vi "Update_Events.vi"(8 "Status/Errors in":refnum<vi>, 9 "Events for screen":refnum<queue>, 10 "Control Parameters [] in":T15[](array[typedef]) {"Aux Byte Value" format="%02x"; "Max Real Value" format="%#_6e"; "Min Real Value" format="%#_6e"; "dReal/dByte" format="%#_6e"; "Byte Value" format="%02x"; "Identifier" format="%02x"}, 11 "Main parameters in":T1={"Mode"={"Mode"=enum."Dialog", "Expert?"=FALSE, "Dialog?"=FALSE}, "Stop loop"={"Settings changed?"=FALSE, "Stop?"=refnum}, "Send message"={"Send mode"=enum."Get parameters", "Set parameter list"=0, "Get parameter list"=0, "Reset device"=0, "Length set settings message"=0, "Reset buttons?"=FALSE, "Reset Master?"=enum."General"}, "Write settings"={"Options"=enum."File 1"}, "Settings state"={"MAS locked?"=refnum, "SLV locked?"=refnum}, "Button refs"={"Stop program"=refnum, "Save settings"=refnum, "DAQ mode"=refnum, "Reset settings"=refnum, "Apply settings"=refnum, "Reset MAS"=refnum, "Reset SLV"=refnum, "Local DBase?"=refnum, "Last value DBase"=FALSE, "Database"=refnum, "Calibration"=refnum, "Save settings 2"=refnum}, "Update screen"={"Detector number"=0, "Hardware"=enum."None"}, "Files"={"Path config file"=path "", "Path def. ini file"=path "", "Path ini file 1"=path "", "Path ini file 2"=path "", "Path RBF file"=path ""}, "DB connection"={"connection reference"=refnum, "Connected?"=refnum, "ODBC Name"=""}, "Status_id"=refnum, "Time difference"=refnum, "Satellites"=refnum, "Alignment parameters"=refnum, "Page Statistics 2"=refnum, "Database"=refnum, "Page Statistics"=refnum} {"Update screen"."Detector number" format="%#.0f"; "Send message"."Reset device" format="%x"; "Send message"."Get parameter list" format="%x"; "Send message"."Set parameter list" format="%x"}) -> (0 "Status/Errors out":refnum<vi>, 2 "Control Parameters [] out":T15[](array[typedef]) {"Aux Byte Value" format="%02x"; "Max Real Value" format="%#_6e"; "Min Real Value" format="%#_6e"; "dReal/dByte" format="%#_6e"; "Byte Value" format="%02x"; "Identifier" format="%02x"}, 3 "Main parameters out":T1={"Mode"={"Mode"=enum."Dialog", "Expert?"=FALSE, "Dialog?"=FALSE}, "Stop loop"={"Settings changed?"=FALSE, "Stop?"=refnum}, "Send message"={"Send mode"=enum."Get parameters", "Set parameter list"=0, "Get parameter list"=0, "Reset device"=0, "Length set settings message"=0, "Reset buttons?"=FALSE, "Reset Master?"=enum."General"}, "Write settings"={"Options"=enum."File 1"}, "Settings state"={"MAS locked?"=refnum, "SLV locked?"=refnum}, "Button refs"={"Stop program"=refnum, "Save settings"=refnum, "DAQ mode"=refnum, "Reset settings"=refnum, "Apply settings"=refnum, "Reset MAS"=refnum, "Reset SLV"=refnum, "Local DBase?"=refnum, "Last value DBase"=FALSE, "Database"=refnum, "Calibration"=refnum, "Save settings 2"=refnum}, "Update screen"={"Detector number"=0, "Hardware"=enum."None"}, "Files"={"Path config file"=path "", "Path def. ini file"=path "", "Path ini file 1"=path "", "Path ini file 2"=path "", "Path RBF file"=path ""}, "DB connection"={"connection reference"=refnum, "Connected?"=refnum, "ODBC Name"=""}, "Status_id"=refnum, "Time difference"=refnum, "Satellites"=refnum, "Alignment parameters"=refnum, "Page Statistics 2"=refnum, "Database"=refnum, "Page Statistics"=refnum} {"Update screen"."Detector number" format="%#.0f"; "Send message"."Reset device" format="%x"; "Send message"."Get parameter list" format="%x"; "Send message"."Set parameter list" format="%x"}, 4 "Updated?":bool)   [LabVIEW 2013]
uses:
  Controls/Control_Parameters.ctl
  Controls/Master.ctl
  Controls/Main_Parameters.ctl
  Controls/Mode.ctl
  Controls/Stop_Loop.ctl
  Controls/Send_Message.ctl
  Controls/Send_Message_Mode.ctl
  Controls/Write_Settings.ctl
  Controls/Write_Settings_Options.ctl
  Controls/Settings_State.ctl
  Controls/Button_Refs.ctl
  Controls/Update_Screen.ctl
  Controls/Files.ctl
  Controls/DB_Connection.ctl
  database/Connection.llb/Conn ObjectReference.ctl
  Controls/Status_Errors_Elements.ctl
  Controls/Get_Set_Statistics_Options2.ctl
  Controls/TabPage_Events.ctl
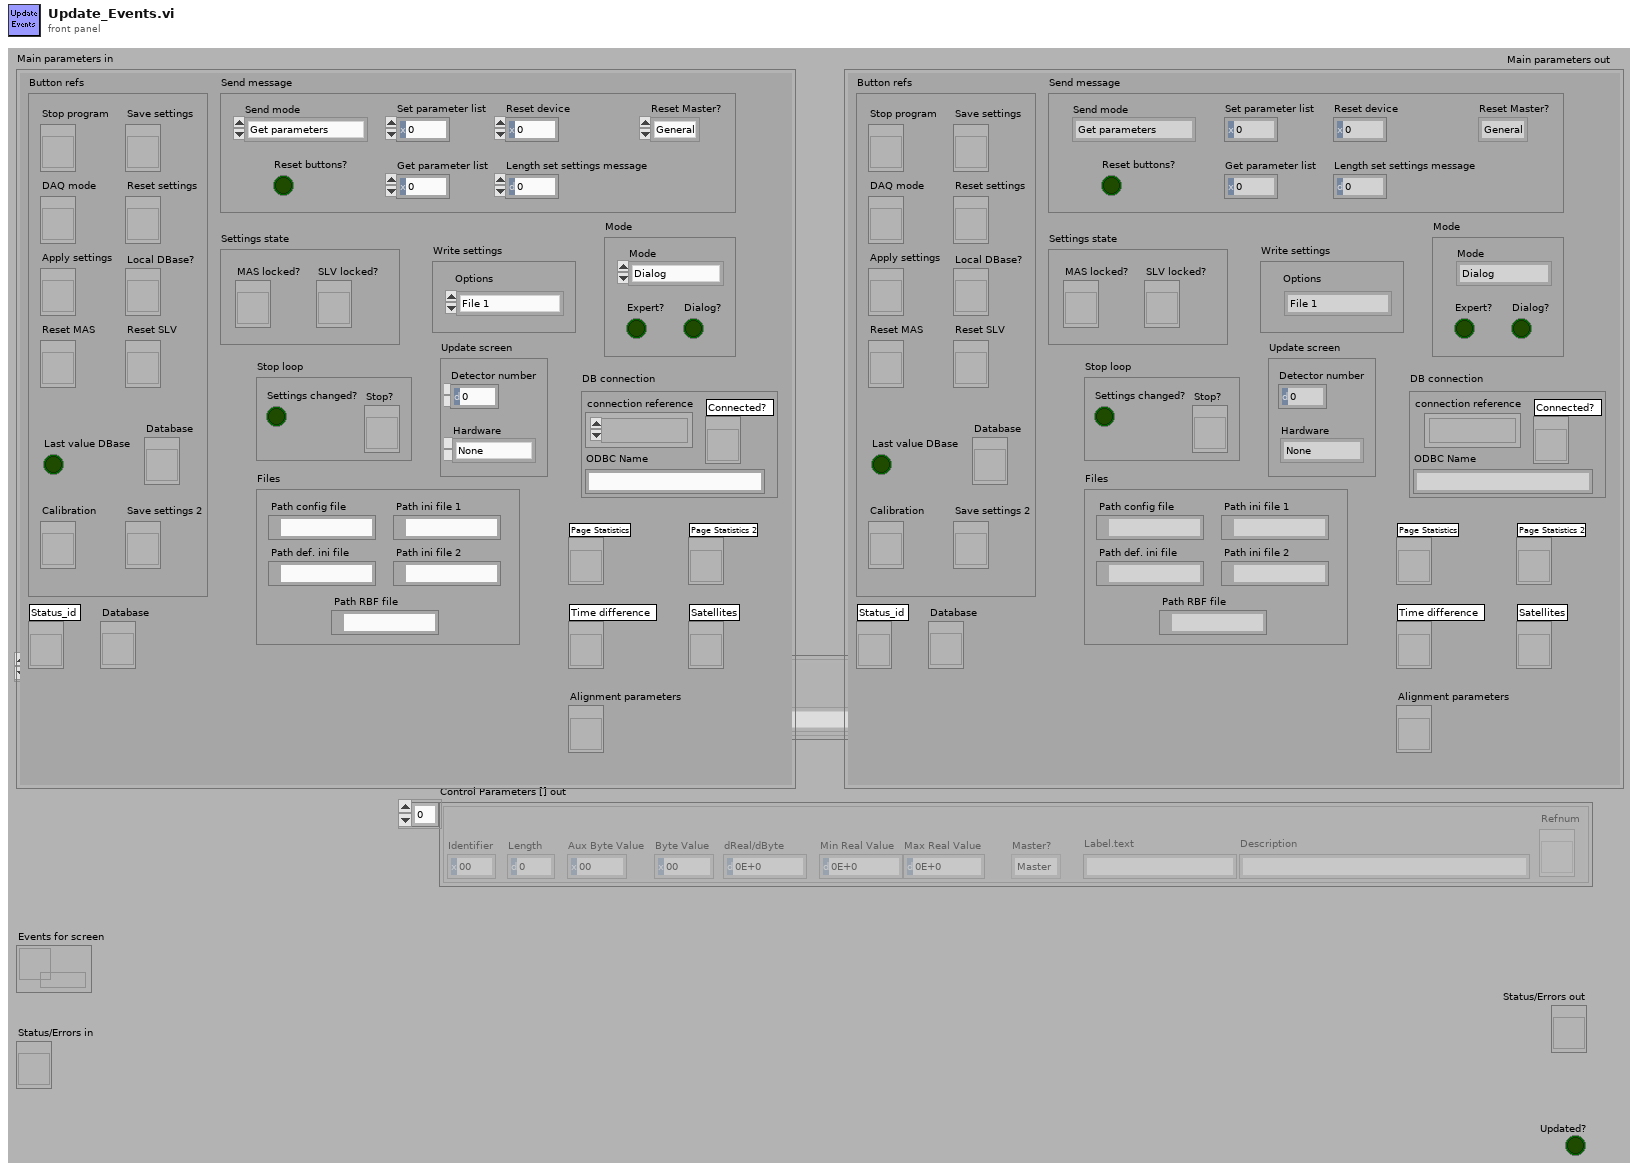
[diagram p1: front panel]
types:
  T1 = typedef "Main_Parameters.ctl" = cluster{"Mode":T2, "Stop loop":T3, "Send message":T4, "Write settings":T7, "Settings state":T9, "Button refs":T10, "Update screen":T11, "Files":T12, "DB connection":T13, "Status_id":refnum<vi>, "Time difference":refnum<vi>, "Satellites":refnum<vi>, "Alignment parameters":refnum<vi>, "Page Statistics 2":refnum<vi>, "Database":refnum<vi>, "Page Statistics":refnum<vi>}
  T2 = typedef "Mode.ctl" = cluster{"Mode":enum8{"Stop", "Dialog", "Hisparc II", "Hisparc II DAQ", "Alignment"}, "Expert?":bool, "Dialog?":bool}
  T3 = typedef "Stop_Loop.ctl" = cluster{"Settings changed?":bool, "Stop?":refnum<vi>}
  T4 = typedef "Send_Message.ctl" = cluster{"Send mode":T5, "Set parameter list":u8, "Get parameter list":u8, "Reset device":u8, "Length set settings message":i32, "Reset buttons?":bool, "Reset Master?":T6}
  T5 = typedef "Send_Message_Mode.ctl" = enum16{"Get parameters", "Set parameters", "From front panel", "From parameters", "Reset device", "Alignment"}
  T6 = typedef "Master.ctl" = enum16{"Master", "Slave", "General"}
  T7 = typedef "Write_Settings.ctl" = cluster{"Options":T8}
  T8 = typedef "Write_Settings_Options.ctl" = enum16{"File 1", "File 2", "Alignment", "Reset"}
  T9 = typedef "Settings_State.ctl" = cluster{"MAS locked?":refnum<vi>, "SLV locked?":refnum<vi>}
  T10 = typedef "Button_Refs.ctl" = cluster{"Stop program":refnum<vi>, "Save settings":refnum<vi>, "DAQ mode":refnum<vi>, "Reset settings":refnum<vi>, "Apply settings":refnum<vi>, "Reset MAS":refnum<vi>, "Reset SLV":refnum<vi>, "Local DBase?":refnum<vi>, "Last value DBase":bool, "Database":refnum<vi>, "Calibration":refnum<vi>, "Save settings 2":refnum<vi>}
  T11 = typedef "Update_Screen.ctl" = cluster{"Detector number":u16, "Hardware":enum8{"None", "HiSPARC I", "HiSPARC II", "HiSPARC III", "Unknown"}}
  T12 = typedef "Files.ctl" = cluster{"Path config file":path, "Path def. ini file":path, "Path ini file 1":path, "Path ini file 2":path, "Path RBF file":path}
  T13 = typedef "DB_Connection.ctl" = cluster{"connection reference":T14, "Connected?":refnum<vi>, "ODBC Name":string}
  T14 = typedef "Conn ObjectReference.ctl" = refnum<k1>
  T15 = typedef "Control_Parameters.ctl" = cluster{"Identifier":u8, "Length":u16, "Byte Value":u32, "dReal/dByte":dbl, "Min Real Value":dbl, "Max Real Value":dbl, "Master?":T6, "Label.text":string, "Description":string, "Refnum":refnum<vi>, "Aux Byte Value":u32}
  T16 = typedef "TabPage_Events.ctl" = cluster{"Det_Numb":u16, "GPS_Timestamp":string, "Trigger_Pattern":cluster{"Master ch. 1 lower threshold":bool, "Master ch. 1 higher threshold":bool, "Master ch. 2 lower threshold":bool, "Master ch. 2 higher threshold":bool, "Slave ch. 1 lower threshold":bool, "Slave ch. 1 higher threshold":bool, "Slave ch. 2 lower threshold":bool, "Slave ch. 2 higher threshold":bool, "External trigger":bool, "Slave present?":bool, "Ch. 1 low comparator master":bool, "Ch. 1 high comparator master":bool, "Ch. 2 low comparator master":bool, "Ch. 2 high comparator master":bool, "Ch. 1 low comparator slave":bool, "Ch. 1 high comparator slave":bool, "Ch. 2 low comparator slave":bool, "Ch. 2 high comparator slave":bool}, "Traces":dbl[][], "MAS_Status_Events":bool, "MAS_Vers_Numb":string, "SLV_Status_Events":bool, "SLV_Vers_Numb":string, "DBase_connected?":bool, "MAS_GPS_Long":dbl, "MAS_GPS_Lat":dbl, "MAS_GPS_Alt":dbl, "Hardware":enum8{"None", "HiSPARC I", "HiSPARC II", "HiSPARC III", "Unknown"}}
  T17 = typedef "Get_Set_Statistics_Options2.ctl" = enum16{"Get", "Set"}
  T18 = typedef "Status_Errors_Elements.ctl" = enum16{"Default", "Errors", "Master status", "Slave status", "Master connected?", "Slave connected?", "Master GPS on board?", "Slave GPS on board?", "Master: slave detected?", "Slave: slave detected?", "Last message from master", "Last message from slave", "Master temperature", "GPS settings correct?"}
  T19 = typedef "Event_Statistics.ctl" = cluster{"Baseline 1":i16, "Baseline 2":i16, "Number of peaks 1":i16, "Number of peaks 2":i16, "Pulse height 1":i16, "Pulse height 2":i16, "Integral 1":i32, "Integral 2":i32, "Standard deviation 1":i16, "Standard deviation 2":i16, "Length":i32, "Time difference":u32}
  T20 = cluster{"Master ch. 1 lower threshold":bool, "Master ch. 1 higher threshold":bool, "Master ch. 2 lower threshold":bool, "Master ch. 2 higher threshold":bool, "Slave ch. 1 lower threshold":bool, "Slave ch. 1 higher threshold":bool, "Slave ch. 2 lower threshold":bool, "Slave ch. 2 higher threshold":bool, "External trigger":bool, "Slave present?":bool, "Ch. 1 low comparator master":bool, "Ch. 1 high comparator master":bool, "Ch. 2 low comparator master":bool, "Ch. 2 high comparator master":bool, "Ch. 1 low comparator slave":bool, "Ch. 1 high comparator slave":bool, "Ch. 2 low comparator slave":bool, "Ch. 2 high comparator slave":bool}
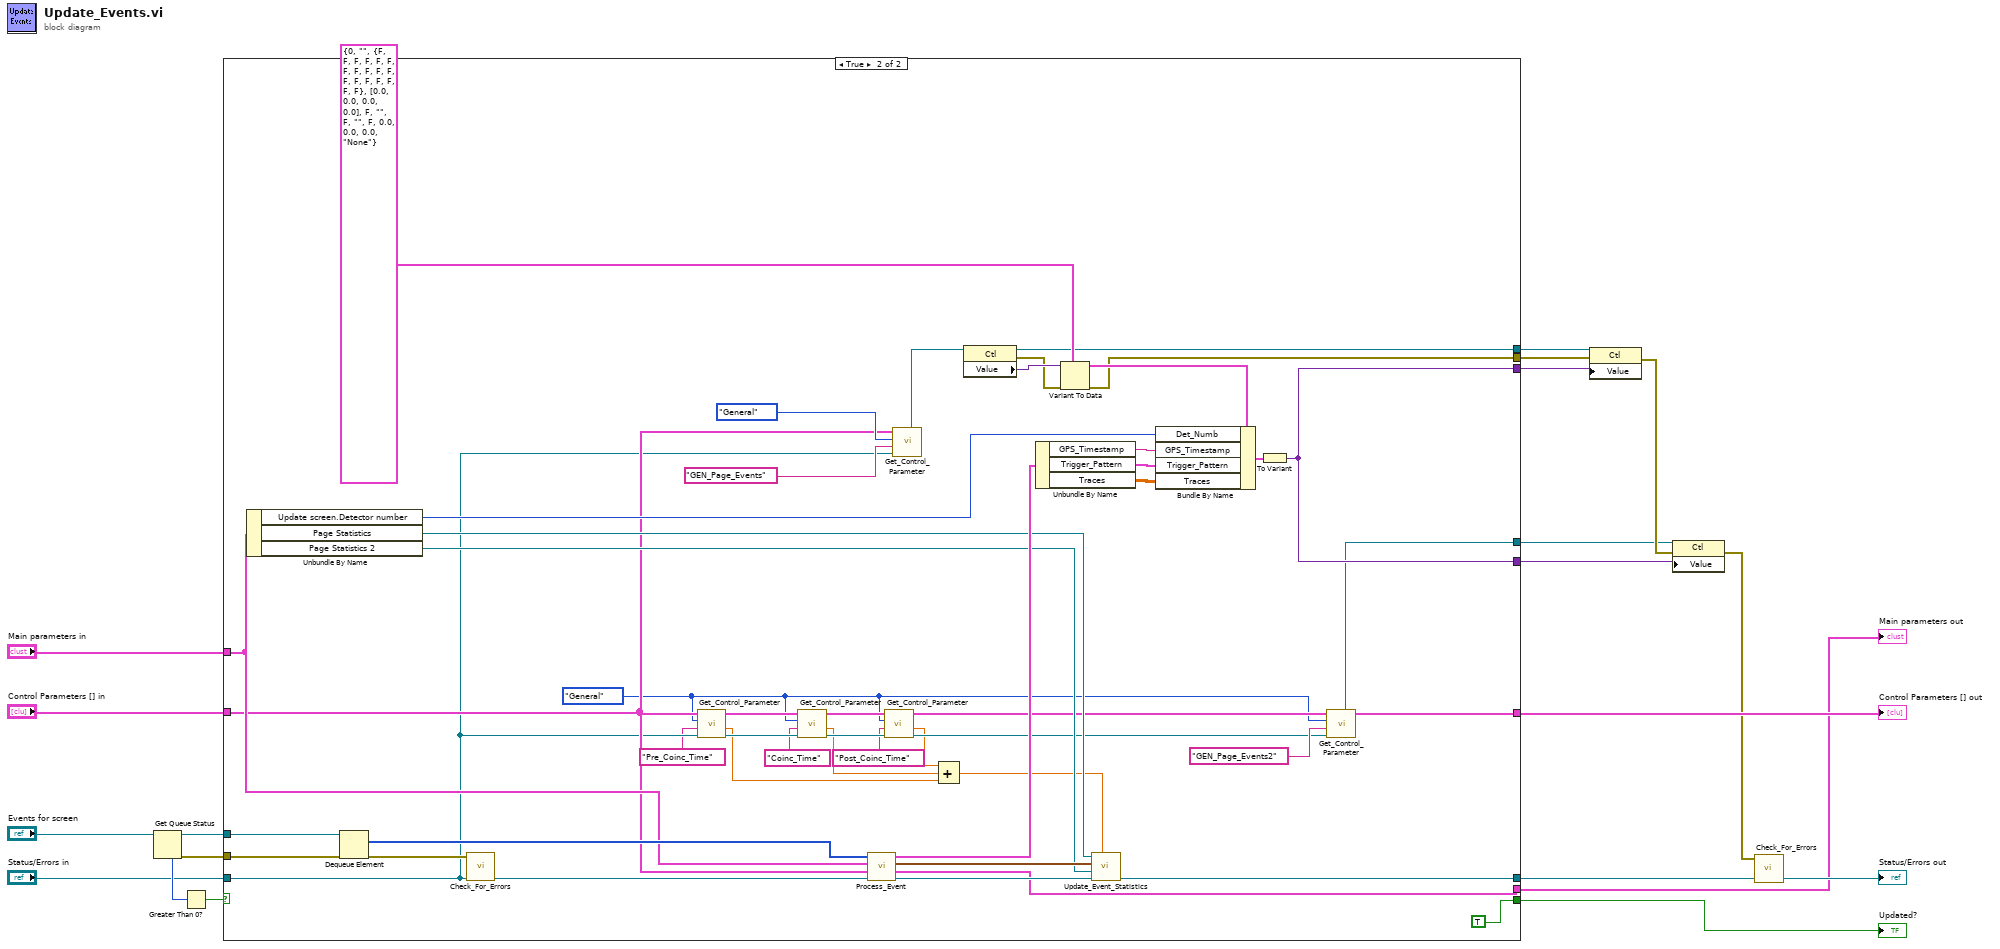
[diagram p0: block diagram]
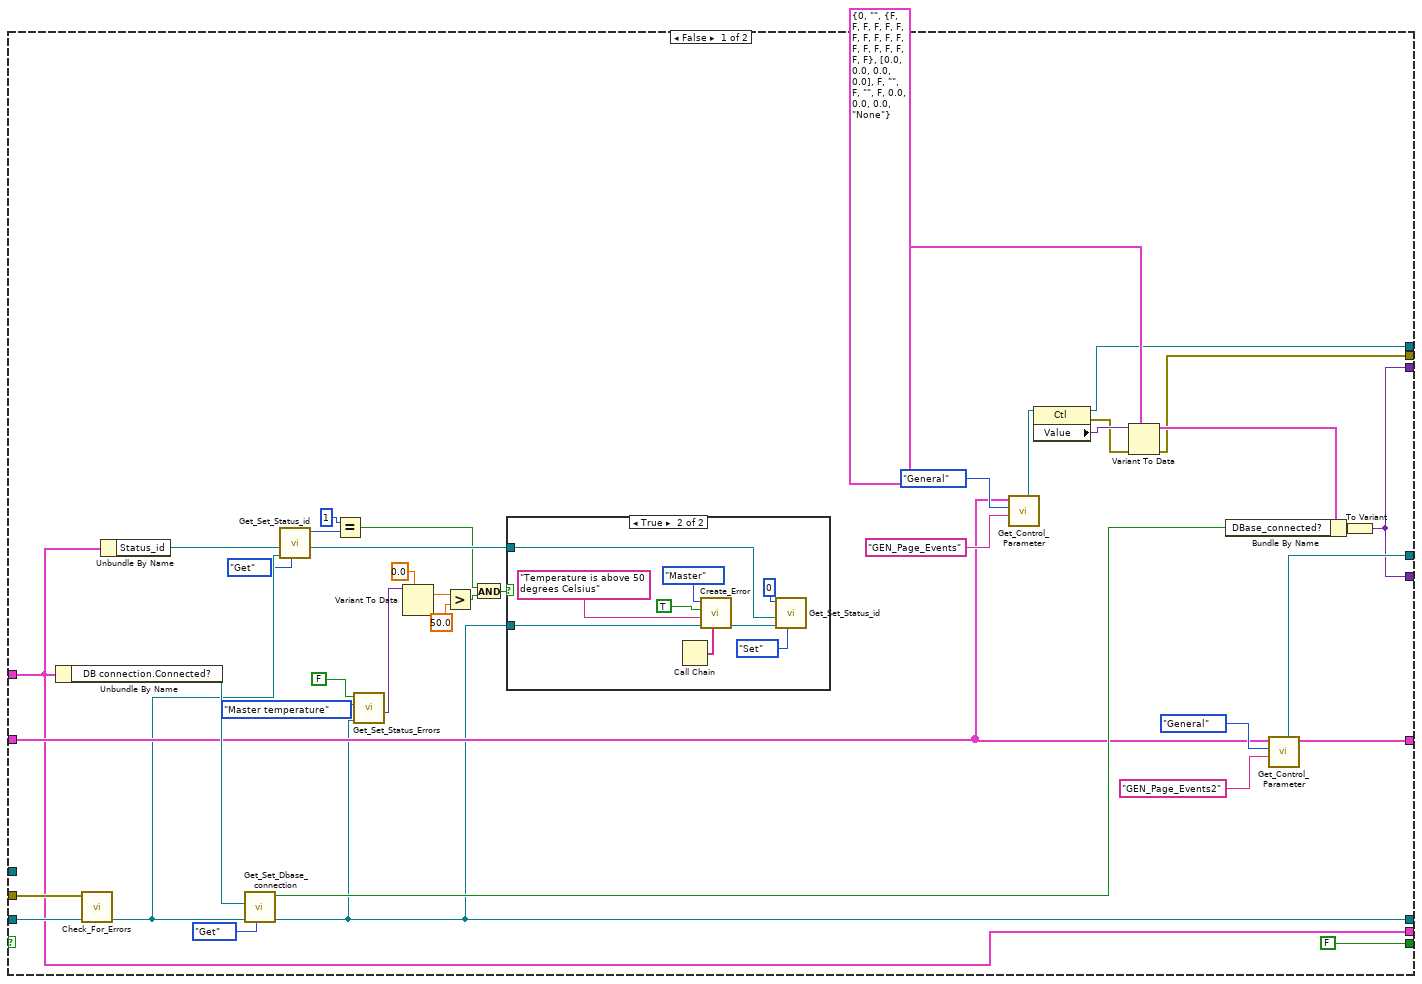
[diagram p2: hidden frame]
diagram:
  n1 = Get Queue Status(queue="Events for screen") -> (queue out=w18:refnum<queue>, error out=w17:errorcluster, # elements in queue=w15:i32)  [unwired: 1 in, 6 out]
  n2 = Greater Than 0?(x=w15) -> (x > 0?=w16:bool)
  n3 = case shown="True" w16 {
    tunnel: [w41 w111] -> w19
    tunnel: [w32 w86] -> w11
    tunnel: "Main parameters in" -> [w29 w84]
    tunnel: "Control Parameters [] in" -> [w42 w83]
    tunnel: w18 -> [_ w100]
    tunnel: w17 -> [w57 w98]
    tunnel: "Status/Errors in" -> [w56 w79]
    tunnel: [FALSE TRUE] -> w10
    tunnel: [w37 w90] -> w6
    tunnel: [w37 w90] -> w5
    tunnel: [w38 w89] -> w4
    tunnel: [w39 w88] -> w3
    tunnel: [w40 w87] -> w2
    tunnel: [w29 w85] -> w1
    frame False {
      n4 = Unbundle By Name(w29) -> ("DB connection.Connected?"=w55:refnum<vi>)
      n5 = call "Check_For_Errors.vi"("Status/Errors in"=w56, "error in"=w57) -> ("Status/Errors out"=w24:refnum<vi>)  [unwired: 9 out]
      n6 = Unbundle By Name(w29) -> ("Status_id"=w25:refnum<vi>)
      n7 = call "Get_Set_Dbase_connection.vi"("Get/Set"=Get_Set_Statistics_Options2."Get", "Status/Errors in"=w24, "Connected? in"=w55) -> ("Status/Errors out"=w32:refnum<vi>, "Value out"=w45:bool)  [unwired: 1 in, 6 out]
      n8 = call "Get_Set_Status_id.vi"("Get/Set"=Get_Set_Statistics_Options2."Get", "Status/Errors in"=w24, "Status_id"=w25) -> ("Status_out"=w26:refnum<vi>, "Value out"=w22:u8)  [unwired: 1 in, 6 out]
      n9 = Equal?(x=u8 1, y=w22) -> (x = y?=w20:bool)
      n10 = call "Get_Set_Status_Errors.vi"("Status/Errors in"=w32, "Element"=Status_Errors_Elements."Master temperature", "Set?"=FALSE) -> ("Value out"=w34:variant)  [unwired: 1 in, 7 out]
      n11 = Variant To Data(type=sgl 0.0 ("y"), Variant=w34) -> (data=w30:sgl)  [unwired: 1 in, 1 out]
      n12 = Greater?(x=w30, y=sgl 50.0) -> (0:w27:bool)
      n13 = And(x=w20, y=w27) -> (x .and. y?=w28:bool)
      n14 = case shown="True" w28 {
        tunnel: w32 -> [_ w65]
        tunnel: w26 -> [_ w60]
        frame False {
        }
        frame True {
          n15 = Call Chain() -> (call chain=w67:string[])
          n16 = call "Create_Error.vi"("Call chain"=w67, "Status/Errors in"=w65, "HiSPARC error"="Temperature is above 50 degrees Celsius", "Warning? (false)"=TRUE, "Master?"=Master."Master") -> ("Status/Errors out"=w62:refnum<vi>)  [unwired: 1 in, 5 out]
          n17 = call "Get_Set_Status_id.vi"("Get/Set"=Get_Set_Statistics_Options2."Set", "Status/Errors in"=w62, "Status_id"=w60, "Value in"=u8 0) -> ()  [unwired: 8 out]
        }
      }
      n18 = call "Get_Control_Parameter.vi"("Label.text in"="GEN_Page_Events", "Master?"=Master."General", "Control Parameters [] in"=w42) -> ("Refnum"=w51:refnum<vi>)  [unwired: 1 in, 7 out]
      n19 = property class="Ctl"(reference=w51) -> (reference out=w39:refnum<vi>, error out=w48:errorcluster, "Value"=w50:variant)  [unwired: 1 in]
      n20 = Variant To Data(error in=w48, type=T16 {"Det_Numb"=0, "GPS_Timestamp"="", "Trigger_Pattern"={"Master ch. 1 lower threshold"=FALSE, "Master ch. 1 higher threshold"=FALSE, "Master ch. 2 lower threshold"=FALSE, "Master ch. 2 higher threshold"=FALSE, "Slave ch. 1 lower threshold"=FALSE, "Slave ch. 1 higher threshold"=FALSE, "Slave ch. 2 lower threshold"=FALSE, "Slave ch. 2 higher threshold"=FALSE, "External trigger"=FALSE, "Slave present?"=FALSE, "Ch. 1 low comparator master"=FALSE, "Ch. 1 high comparator master"=FALSE, "Ch. 2 low comparator master"=FALSE, "Ch. 2 high comparator master"=FALSE, "Ch. 1 low comparator slave"=FALSE, "Ch. 1 high comparator slave"=FALSE, "Ch. 2 low comparator slave"=FALSE, "Ch. 2 high comparator slave"=FALSE}, "Traces"=[[0.0, 0.0], [0.0, 0.0]], "MAS_Status_Events"=FALSE, "MAS_Vers_Numb"="", "SLV_Status_Events"=FALSE, "SLV_Vers_Numb"="", "DBase_connected?"=FALSE, "MAS_GPS_Long"=0.0, "MAS_GPS_Lat"=0.0, "MAS_GPS_Alt"=0.0, "Hardware"=enum."None"} ("Event cluster"), Variant=w50) -> (data=w47:T16, error out=w38:errorcluster)
      n21 = Bundle By Name(cluster=w47, "DBase_connected?"=w45) -> (w46:T16)
      n22 = call "Get_Control_Parameter.vi"("Label.text in"="GEN_Page_Events2", "Master?"=Master."General", "Control Parameters [] in"=w42) -> ("Control Parameters [] out"=w41:T15[], "Refnum"=w40:refnum<vi>)  [unwired: 1 in, 6 out]
      n23 = To Variant(anything=w46) -> (Variant=w37:variant)
    }
    frame True {
      w75 = Master."General" ("Master?")
      n24 = Unbundle By Name(w84) -> ("Update screen.Detector number"=w93:u16, "Page Statistics"=w92:refnum<vi>, "Page Statistics 2"=w91:refnum<vi>)
      n25 = Dequeue Element(queue=w100, error in (no error)=w98) -> (element=w99:u8[], error out=w97:errorcluster)  [unwired: 3 out]
      n26 = call "Check_For_Errors.vi"("Status/Errors in"=w79, "error in"=w97) -> ("Status/Errors out"=w114:refnum<vi>)  [unwired: 9 out]
      n27 = call "Get_Control_Parameter.vi"("Status/Errors in"=w79, "Label.text in"="Pre_Coinc_Time", "Master?"=w75, "Control Parameters [] in"=w83) -> ("Status/Errors out"=w78:refnum<vi>, "Real Value"=w71:dbl, "Control Parameters [] out"=w82:T15[])  [unwired: 5 out]
      n28 = call "Get_Control_Parameter.vi"("Status/Errors in"=w78, "Label.text in"="Coinc_Time", "Master?"=w75, "Control Parameters [] in"=w82) -> ("Status/Errors out"=w77:refnum<vi>, "Real Value"=w70:dbl, "Control Parameters [] out"=w81:T15[])  [unwired: 5 out]
      n29 = call "Process_Event.vi"("Status/Errors in"=w114, "Control Parameters [] in"=w83, "Main parameters in"=w84, "Event array"=w99) -> ("Status/Errors out"=w95:refnum<vi>, "Main parameters out"=w85:T1, "Event statistics"=w94:T19[], "Event cluster"=w104:T16)  [unwired: 4 out]
      n30 = call "Get_Control_Parameter.vi"("Status/Errors in"=w77, "Label.text in"="Post_Coinc_Time", "Master?"=w75, "Control Parameters [] in"=w81) -> ("Status/Errors out"=w76:refnum<vi>, "Real Value"=w69:dbl, "Control Parameters [] out"=w80:T15[])  [unwired: 5 out]
      n31 = call "Get_Control_Parameter.vi"("Status/Errors in"=w79, "Label.text in"="GEN_Page_Events", "Master?"=Master."General", "Control Parameters [] in"=w83) -> ("Refnum"=w110:refnum<vi>)  [unwired: 7 out]
      n32 = Compound Arithmetic op=ADD(w69, w70, w71) -> (w68:dbl)
      n33 = property class="Ctl"(reference=w110) -> (reference out=w88:refnum<vi>, error out=w107:errorcluster, "Value"=w109:variant)  [unwired: 1 in]
      n34 = Unbundle By Name(w104) -> ("GPS_Timestamp"=w103:string, "Trigger_Pattern"=w102:T20, "Traces"=w101:dbl[][])
      n35 = Variant To Data(error in=w107, type=T16 {"Det_Numb"=0, "GPS_Timestamp"="", "Trigger_Pattern"={"Master ch. 1 lower threshold"=FALSE, "Master ch. 1 higher threshold"=FALSE, "Master ch. 2 lower threshold"=FALSE, "Master ch. 2 higher threshold"=FALSE, "Slave ch. 1 lower threshold"=FALSE, "Slave ch. 1 higher threshold"=FALSE, "Slave ch. 2 lower threshold"=FALSE, "Slave ch. 2 higher threshold"=FALSE, "External trigger"=FALSE, "Slave present?"=FALSE, "Ch. 1 low comparator master"=FALSE, "Ch. 1 high comparator master"=FALSE, "Ch. 2 low comparator master"=FALSE, "Ch. 2 high comparator master"=FALSE, "Ch. 1 low comparator slave"=FALSE, "Ch. 1 high comparator slave"=FALSE, "Ch. 2 low comparator slave"=FALSE, "Ch. 2 high comparator slave"=FALSE}, "Traces"=[[0.0, 0.0], [0.0, 0.0]], "MAS_Status_Events"=FALSE, "MAS_Vers_Numb"="", "SLV_Status_Events"=FALSE, "SLV_Vers_Numb"="", "DBase_connected?"=FALSE, "MAS_GPS_Long"=0.0, "MAS_GPS_Lat"=0.0, "MAS_GPS_Alt"=0.0, "Hardware"=enum."None"} ("Event cluster"), Variant=w109) -> (data=w106:T16, error out=w89:errorcluster)
      n36 = call "Update_Event_Statistics.vi"("Total_coincidence_time"=w68, "Status/Errors in"=w95, "Page Statistics 2"=w91, "Event statistics"=w94, "Page Statistics"=w92) -> ("Status/Errors out"=w86:refnum<vi>)  [unwired: 6 out]
      n37 = Bundle By Name(cluster=w106, "Det_Numb"=w93, "GPS_Timestamp"=w103, "Trigger_Pattern"=w102, "Traces"=w101) -> (w105:T16)
      n38 = To Variant(anything=w105) -> (Variant=w90:variant)
      n39 = call "Get_Control_Parameter.vi"("Status/Errors in"=w76, "Label.text in"="GEN_Page_Events2", "Master?"=w75, "Control Parameters [] in"=w80) -> ("Control Parameters [] out"=w111:T15[], "Refnum"=w87:refnum<vi>)  [unwired: 6 out]
    }
  }
  "Control Parameters [] out" <- w19
  "Status/Errors out" <- w11
  "Main parameters out" <- w1
  "Updated?" <- w10
  n40 = property class="Ctl"(reference=w3, error in=w4, "Value"=w5) -> (error out=w7:errorcluster)  [unwired: 1 out]
  n41 = property class="Ctl"(reference=w2, error in=w7, "Value"=w6) -> (error out=w8:errorcluster)  [unwired: 1 out]
  n42 = call "Check_For_Errors.vi"("error in"=w8) -> ()  [unwired: 1 in, 10 out]
